vi "Get BackColor.vi"(8 "error in (no error)":errorcluster, 11 "View in":refnum<class "Cell View.lvclass">) -> (0 "error out":errorcluster, 2 "Color.lvclass":refnum<class "Color.lvclass">, 3 "View out":refnum<class "Cell View.lvclass">)   [LabVIEW 2024, in "Cell View.lvclass"]
uses:
  Cell View.lvclass
  Color/Color.lvclass
  Cell View.lvclass/Cell View.ctl
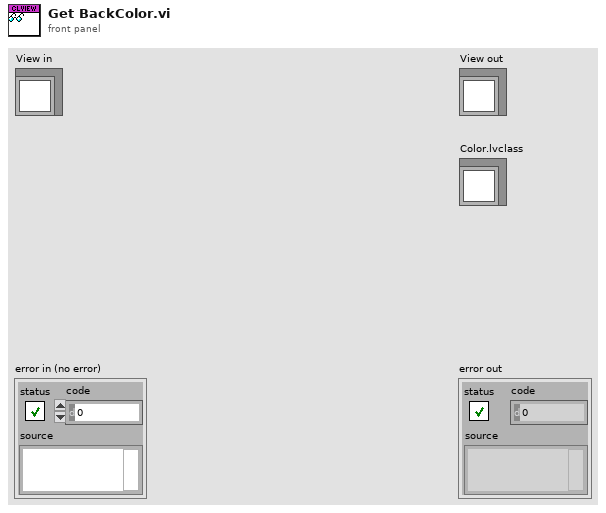
[diagram p1: front panel]
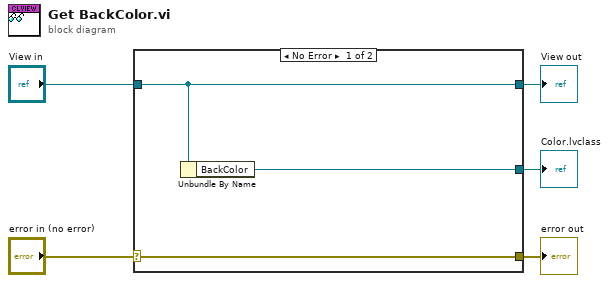
[diagram p0: block diagram]
diagram:
  n1 = case shown="No Error" "error in (no error)" {
    selector: "error in (no error)" -> [w8 w9]
    tunnel: [w8 w9] -> w4
    tunnel: [w7 w10] -> w2
    tunnel: "View in" -> [w7 w10]
    tunnel: [w6 _] -> w1
    frame No Error {
      n2 = Unbundle By Name(w7) -> ("BackColor"=w6:refnum<class "Color.lvclass">)
    }
    frame Error {
    }
  }
  "error out" <- w4
  "View out" <- w2
  "Color.lvclass" <- w1
